vi "RILIS Remote Control.vi"() -> ()   [LabVIEW 2013]
uses:
  Global Variables/Global Stop.vi
panel:
  in  "Open Setup Scanner":bool
  in  "Step Size":i32=100 caption="Max. 500"
  in  "Enable Keyboard Control Button":bool
  in  "Open Scan Coordinator":bool
  in  "Tab Control":T1(tab)
  in  "Display History":i32=500 caption="Values"
  out "NB-TiSa Data vs Time":cluster{cluster{dbl, "Value":dbl}[]}[](graph)
  in  "Clear Time Graph":bool
  out "Wavelength vs. Thick Etalon Position":cluster{cluster{"Value":i32, "Value":dbl}[]}[](graph)
  out "Wavelength vs. Thin Etalon Position":cluster{cluster{"Value":i32, "Value":dbl}[]}[](graph)
  in  "Clear WL vs ThinPos":bool
  out "Power vs. Thick Etalon Position":cluster{cluster{"Value":i32, "Value":dbl}[]}[](graph)
  in  "Clear POW vs ThickPos":bool
  out "Power vs. Thin Etalon Position":cluster{cluster{"Value":i32, "Value":dbl}[]}[](graph)
  in  "Clear POW vs ThinPos":bool
  in  "Clear WL vs ThickPos":bool
  out "WS7 Pattern2 Data":u16[](graph)
  out "WS7 Pattern1 Data":u16[](graph)
  out "DAQ loop counter":i32
  out "Event Loop Counter":i32
  in  "Copy Values":bool
  in  "HELP Button":bool
  in  "Open Linewidth Sweep":bool
  in  "Open Dual Etalon Scanner":bool
  in  "Open Prop Stabilization":bool
  out "Thin Etalon Position":i32
  out "Thick Etalon Position":i32
  in  "Thin Etalon Position Setpoint":i32
  in  "Thick Etalon Position Setpoint":i32
  out "Linewidth":dbl format="%.2f"
  out "Power":dbl format="%.2f"
  in  "Stop":bool
  out "Wavenumber":dbl format="%.4f"
  # "UP, DOWN moves thick etalon\nLEFT, RIGHT moves thin etalon"
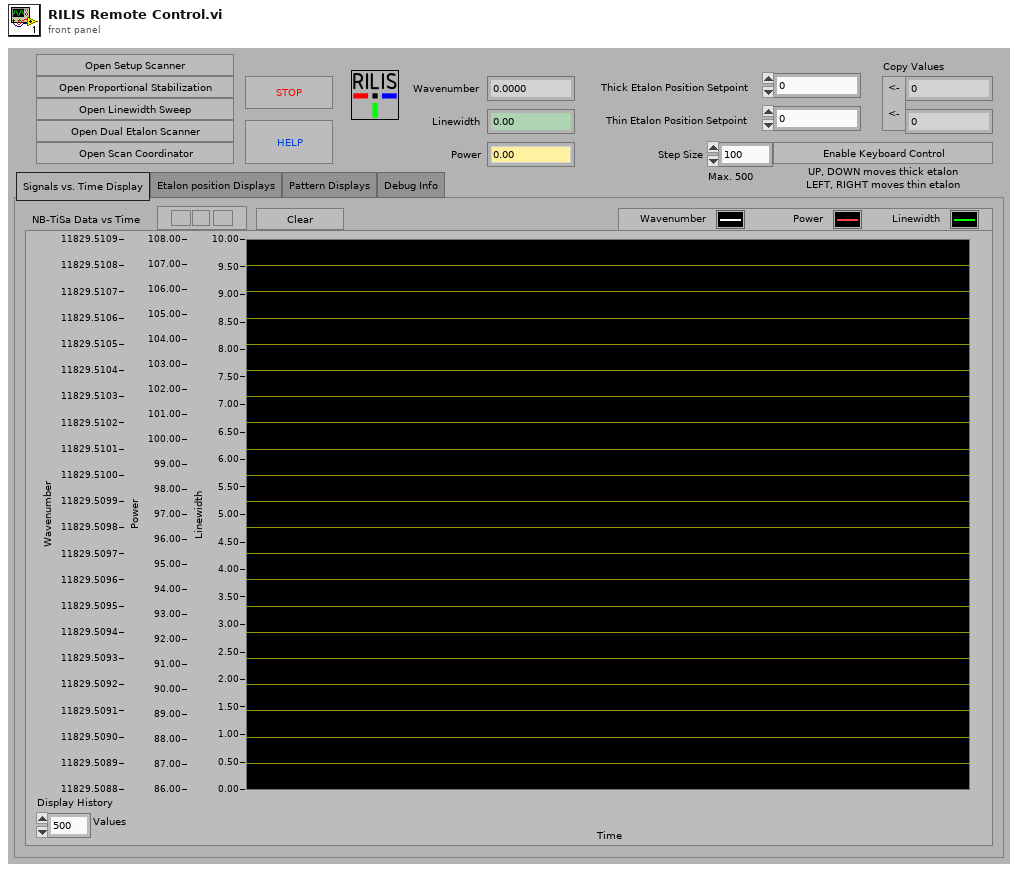
[diagram p1: front panel]
types:
  T1 = enum32{"Signals vs. Time Display", "Etalon position Displays", "Pattern Displays", "Debug Info"}
  T2 = enum32{"Bad", "Idle", "Run top level", "Running"}
  T3 = enum32{"Invalid", "Standard", "Closed", "Hidden", "Minimized", "Maximized"}
  T4 = typedef "eventvkey.ctl" = enum16{"ASCII", "Enter", "Return", "Shift", "Ctrl", "Alt", "Cmd", "Opt", "Caps", "NumLock", "Clear", "Break", "Up", "Down", "Left", "Right", "Insert", "Delete", "Home", "End", "PageUp", "PageDown", "Escape", "Help", "Pause", "ScrollLock", "F1", "F2", "F3", "F4", "F5", "F6", "F7", "F8", "F9", "F10", "F11", "F12", "F13", "F14", "F15", "F16", "F17", "F18", "F19", "F20", "F21", "F22", "F23", "F24", "Play", "VolumeUp", "VolumeDown", "Mute", "Two Byte Char"}
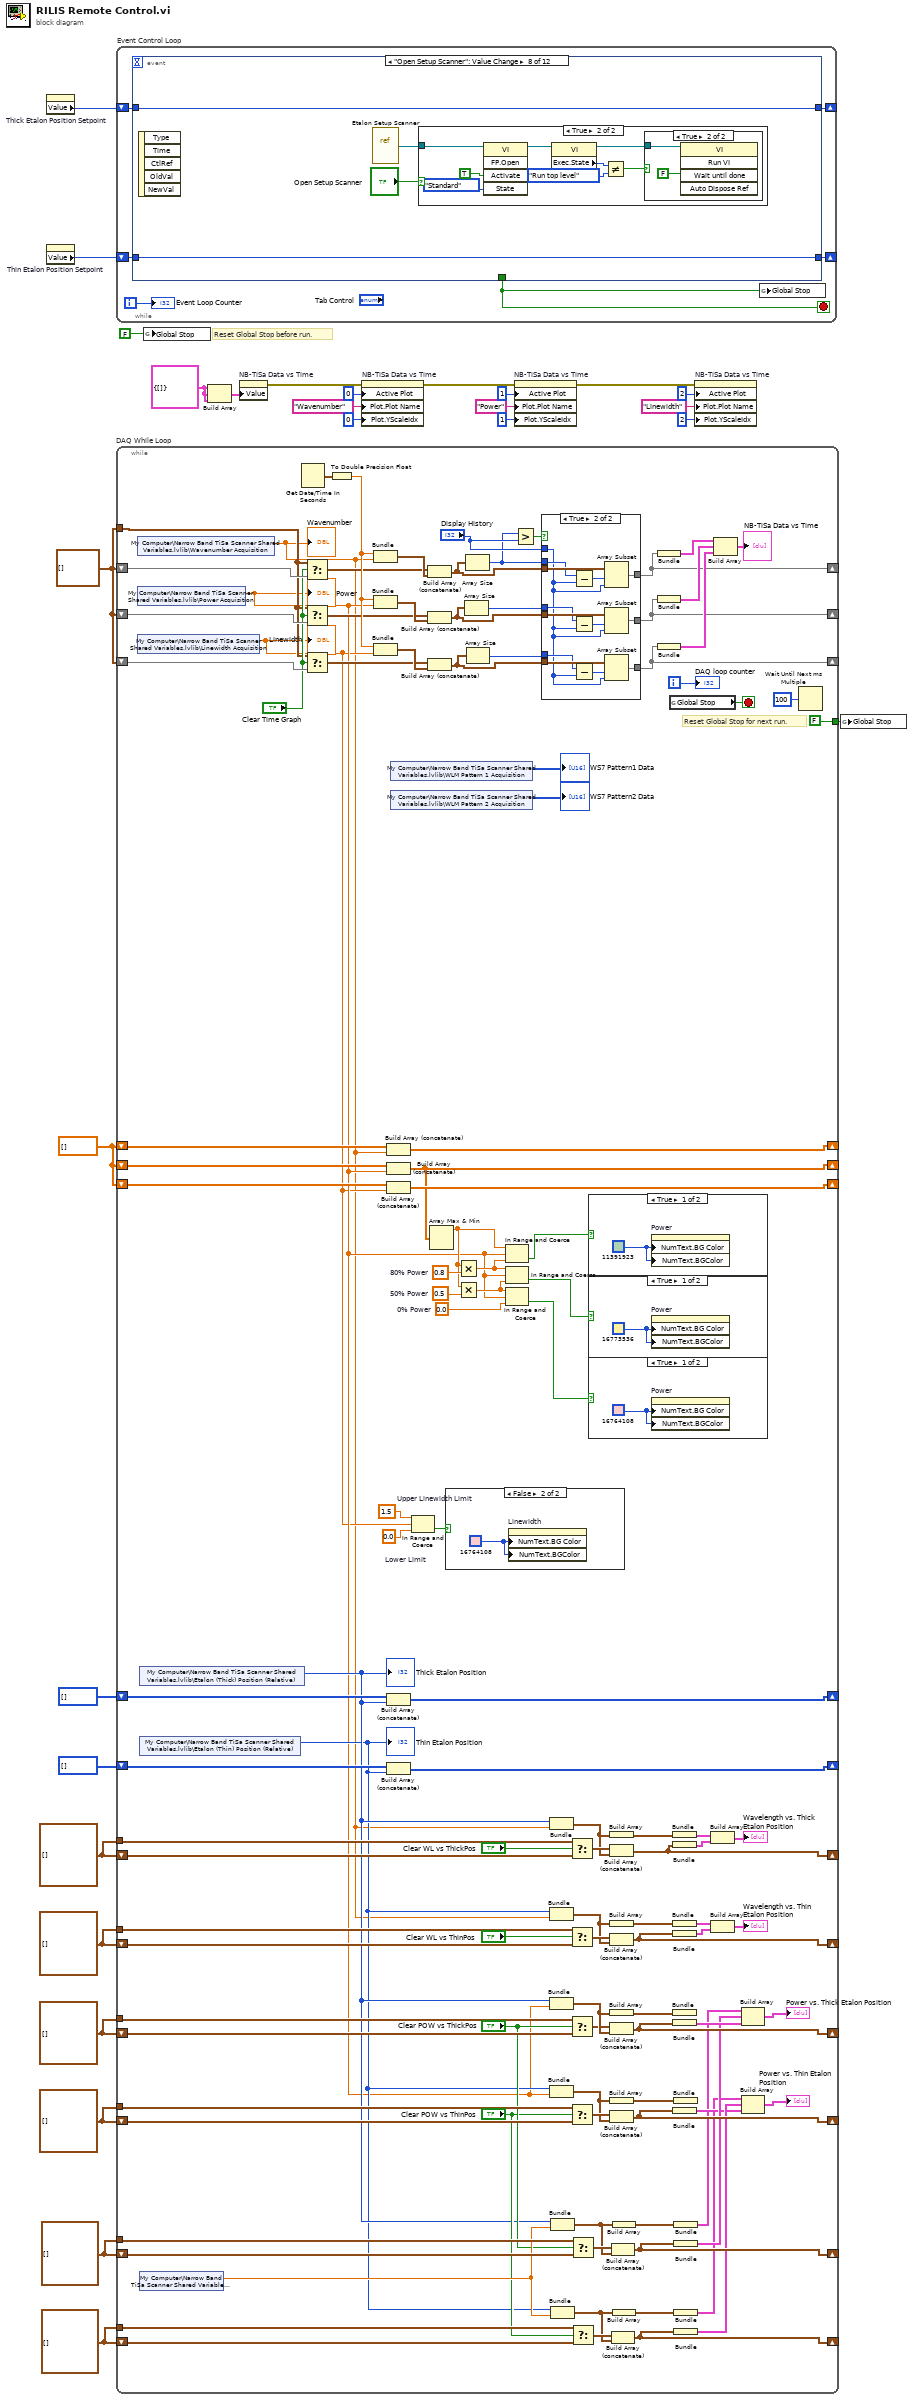
[diagram p0: block diagram]
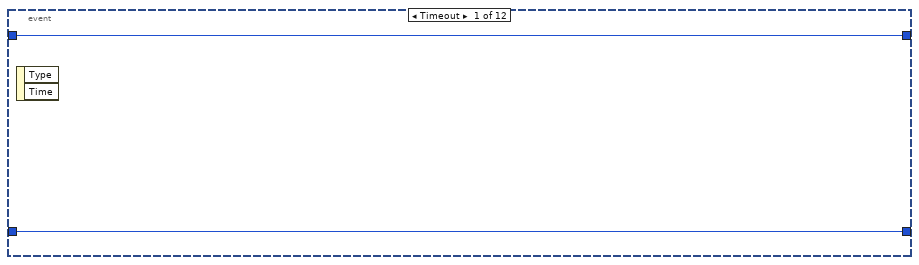
[diagram p2: hidden frame]
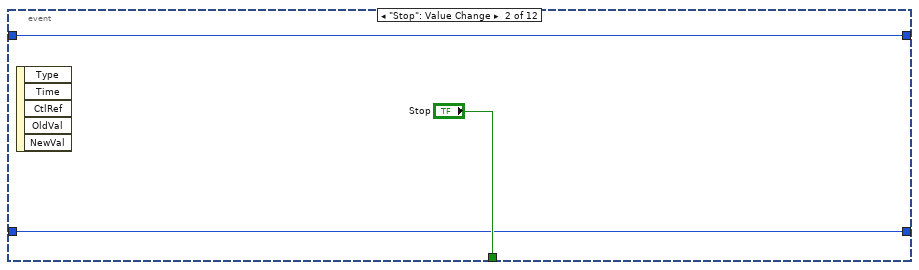
[diagram p3: hidden frame]
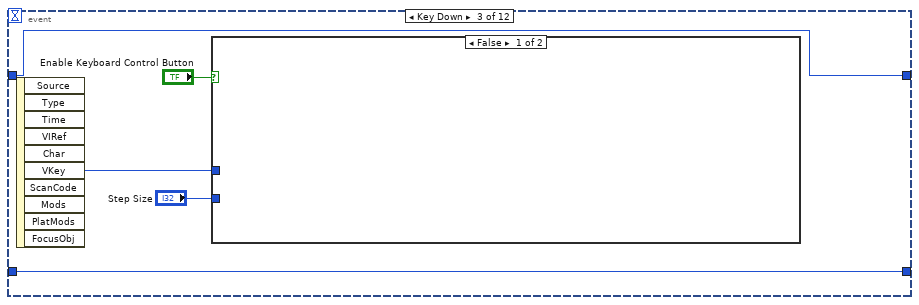
[diagram p4: hidden frame]
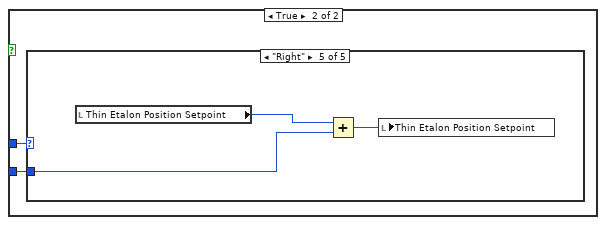
[diagram p5: hidden frame]
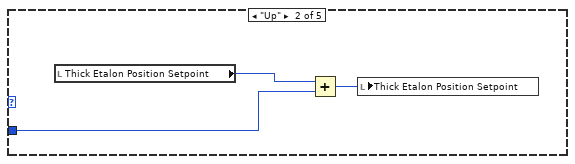
[diagram p7: hidden frame]
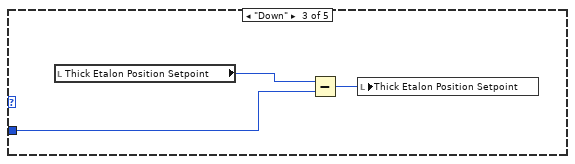
[diagram p8: hidden frame]
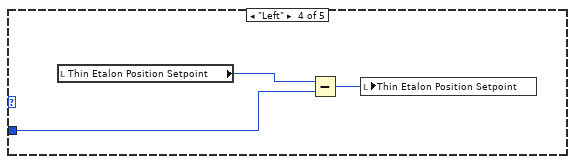
[diagram p9: hidden frame]
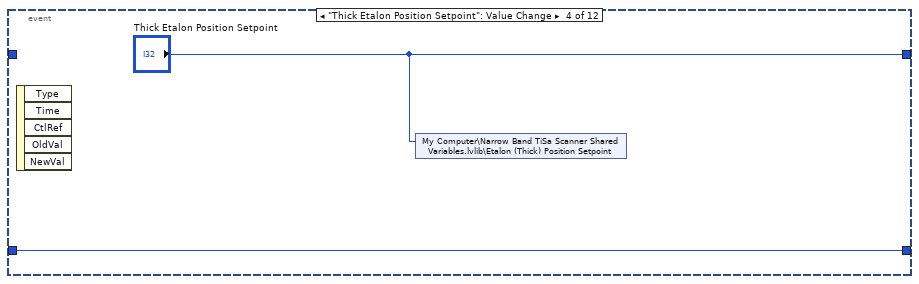
[diagram p10: hidden frame]
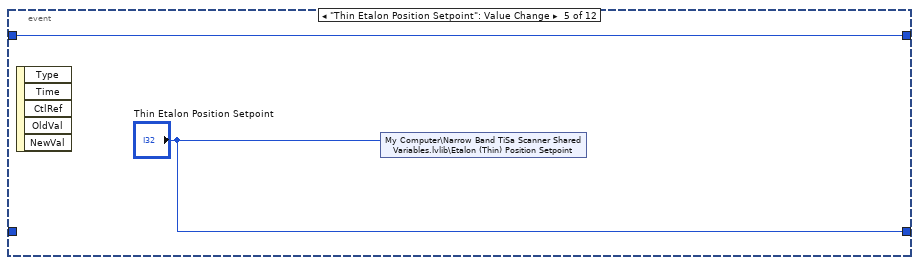
[diagram p11: hidden frame]
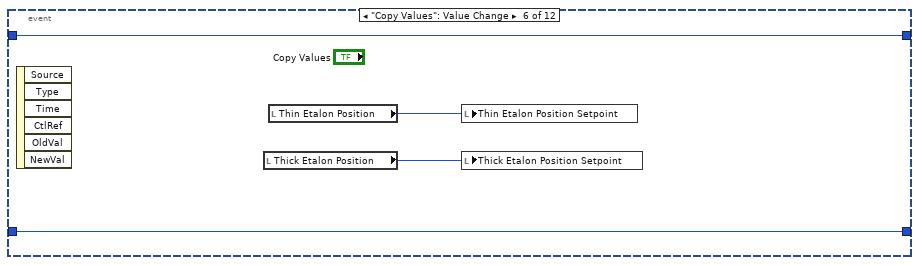
[diagram p12: hidden frame]
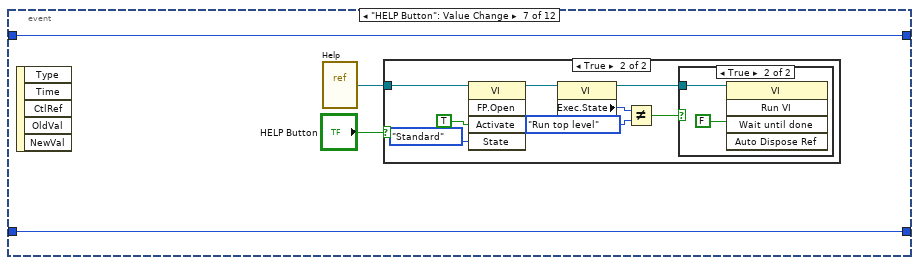
[diagram p13: hidden frame]
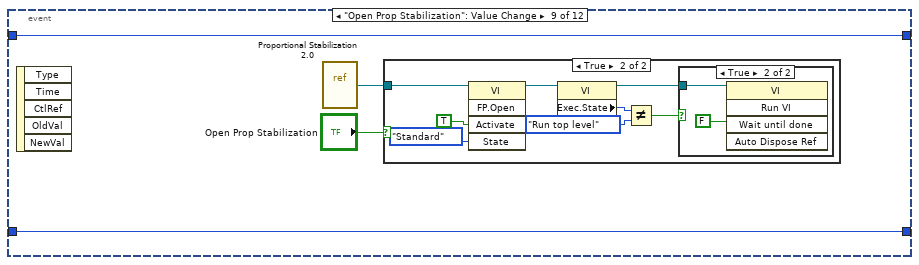
[diagram p18: hidden frame]
diagram:
  w2 = cluster{"Value":i32, "Value":dbl}[] []
  w1 = cluster{"Value":i32, "Value":dbl}[] []
  w3 = dbl[] []
  w6 = cluster{"Value":i32, "Value":dbl}[] []
  w7 = cluster{"Value":i32, "Value":dbl}[] []
  w8 = cluster{"Value":i32, "Value":dbl}[] []
  w9 = cluster{"Value":i32, "Value":dbl}[] []
  w27 = cluster{cluster{dbl, "Value":dbl}[]} {[]} ("output cluster")
  w12 = cluster{dbl, "Value":dbl}[] []
  # "Reset Global Stop before run."
  n1 = property on="Thick Etalon Position Setpoint" class="DigNum (strict)"() -> ("Value"=w11:i32)  [unwired: 2 in, 2 out]
  n2 = property on="Thin Etalon Position Setpoint" class="DigNum (strict)"() -> ("Value"=w10:i32)  [unwired: 2 in, 2 out]
  n3 = while "DAQ While Loop" {
    shift-right: [w130] -> _
    shift-left: w12 -> [w115]
    shift-right: [w129] -> _
    shift-left: w12 -> [w116]
    shift-right: [w128] -> _
    shift-left: w12 -> [w117]
    tunnel: [FALSE] -> w13
    tunnel: w12 -> [w113]
    shift-right: [w109] -> _
    shift-left: w9 -> [w111]
    shift-right: [w101] -> _
    shift-left: w8 -> [w103]
    tunnel: w9 -> [w105]
    tunnel: w8 -> [w104]
    shift-right: [w93] -> _
    shift-left: w7 -> [w91]
    tunnel: w7 -> [w90]
    shift-right: [w86] -> _
    shift-left: w6 -> [w88]
    tunnel: w6 -> [w89]
    shift-right: [w79] -> _
    shift-left: i32[] [] -> [w82]
    shift-right: [w78] -> _
    shift-left: i32[] [] -> [w81]
    shift-right: [w77] -> _
    shift-left: w3 -> [w80]
    shift-right: [w72] -> _
    shift-left: w3 -> [w71]
    shift-right: [w69] -> _
    shift-left: w3 -> [w70]
    shift-right: [w49] -> _
    shift-left: w1 -> [w51]
    tunnel: w1 -> [w52]
    shift-right: [w56] -> _
    shift-left: w2 -> [w54]
    tunnel: w2 -> [w53]
    i -> [w144]
    stop <- w122 stop-if-true
    w60 = 0.0  # 0% Power
    w63 = 0.5  # 50% Power
    w66 = 0.0  # Lower Limit
    w68 = 0.8  # 80% Power
    w67 = 1.5  # Upper Linewidth Limit
    # "Reset Global Stop for next run."
    n4 = shared-variable "My Computer\\Narrow Band TiSa Scanner Shared Variables.lvlib\\Wavenumber Acquisition"() -> (w29:dbl)  [unwired: 1 in, 1 out]
    "Wavenumber" <- w29
    n5 = shared-variable "My Computer\\Narrow Band TiSa Scanner Shared Variables.lvlib\\Power Acquisition"() -> (w43:dbl)  [unwired: 1 in, 1 out]
    "Power" <- w43
    n6 = shared-variable "My Computer\\Narrow Band TiSa Scanner Shared Variables.lvlib\\Linewidth Acquisition"() -> (w42:dbl)  [unwired: 1 in, 1 out]
    "Linewidth" <- w42
    n7 = shared-variable "My Computer\\Narrow Band TiSa Scanner Shared Variables.lvlib\\Etalon (Thick) Position (Relative)"() -> (w45:i32)  [unwired: 1 in, 1 out]
    "Thick Etalon Position" <- w45
    n8 = shared-variable "My Computer\\Narrow Band TiSa Scanner Shared Variables.lvlib\\Etalon (Thin) Position (Relative)"() -> (w44:i32)  [unwired: 1 in, 1 out]
    "Thin Etalon Position" <- w44
    n9 = shared-variable "My Computer\\Narrow Band TiSa Scanner Shared Variables.lvlib\\Power MPM"() -> (w48:dbl)  [unwired: 1 in, 1 out]
    n10 = Get Date/Time In Seconds() -> (seconds since 1Jan1904=w142:timestamp)
    n11 = Select(t=w113, s="Clear Time Graph", f=w115) -> (s? t:f=w120:cluster{dbl, "Double":dbl}[])
    n12 = Select(t=w113, s="Clear Time Graph", f=w116) -> (s? t:f=w119:cluster{dbl, "Double":dbl}[])
    n13 = Select(t=w113, s="Clear Time Graph", f=w117) -> (s? t:f=w118:cluster{dbl, "Double":dbl}[])
    n14 = To Double Precision Float(number=w142) -> (double precision float=w141:dbl)
    n15 = Bundle(w141, "Double"=w29) -> (w140:cluster{dbl, "Double":dbl})  [unwired: 1 in]
    n16 = Bundle(w141, "Double"=w43) -> (w139:cluster{dbl, "Double":dbl})  [unwired: 1 in]
    n17 = Bundle(w141, "Double"=w42) -> (w138:cluster{dbl, "Double":dbl})  [unwired: 1 in]
    n18 = Build Array (concatenate)(w80, w29) -> (w77:dbl[])
    n19 = Build Array (concatenate)(w70, w43) -> (w69:dbl[])
    n20 = Build Array (concatenate)(w71, w42) -> (w72:dbl[])
    n21 = Build Array (concatenate)(w82, w45) -> (w79:i32[])
    n22 = Build Array (concatenate)(w81, w44) -> (w78:i32[])
    n23 = shared-variable "My Computer\\Narrow Band TiSa Scanner Shared Variables.lvlib\\WLM Pattern 1 Acquisition"() -> (→"WS7 Pattern1 Data":u16[])  [unwired: 1 in, 1 out]
    n24 = shared-variable "My Computer\\Narrow Band TiSa Scanner Shared Variables.lvlib\\WLM Pattern 2 Acquisition"() -> (→"WS7 Pattern2 Data":u16[])  [unwired: 1 in, 1 out]
    n25 = In Range and Coerce(upper limit=w67, x=w42, lower limit=w66) -> (In Range?=w65:bool)  [unwired: 1 out]
    n26 = Build Array (concatenate)(w120, w140) -> (w132:cluster{dbl, "Double":dbl}[])
    n27 = Build Array (concatenate)(w119, w139) -> (w133:cluster{dbl, "Double":dbl}[])
    n28 = Build Array (concatenate)(w118, w138) -> (w131:cluster{dbl, "Double":dbl}[])
    n29 = Array Max & Min(array=w69) -> (max value=w62:dbl)  [unwired: 3 out]
    n30 = case shown="False" w65 {
      frame True {
        w148 = u32 11391923
        n31 = property on="Linewidth" class="DigNum (strict)"("NumText.BG Color"=w148, "NumText.BGColor"=w148) -> ()  [unwired: 2 in, 2 out]
      }
      frame False {
        w149 = u32 16764108
        n32 = property on="Linewidth" class="DigNum (strict)"("NumText.BG Color"=w149, "NumText.BGColor"=w149) -> ()  [unwired: 2 in, 2 out]
      }
    }
    n33 = Multiply(x=w62, y=w68) -> (x*y=w64:dbl)
    n34 = Multiply(x=w62, y=w63) -> (x*y=w61:dbl)
    n35 = Array Size(array=w133) -> (size(s)=w125:i32)
    n36 = Array Size(array=w132) -> (size(s)=w124:i32)
    n37 = Array Size(array=w131) -> (size(s)=w123:i32)
    n38 = In Range and Coerce(upper limit=w62, x=w43, lower limit=w64) -> (In Range?=w59:bool)  [unwired: 1 out]
    n39 = In Range and Coerce(upper limit=w64, x=w43, lower limit=w61) -> (In Range?=w58:bool)  [unwired: 1 out]
    n40 = In Range and Coerce(upper limit=w61, x=w43, lower limit=w60) -> (In Range?=w57:bool)  [unwired: 1 out]
    n41 = Greater?(x=w124, y="Display History") -> (0:w126:bool)
    n42 = case shown="True" w126 {
      tunnel: w133 -> [w151 w165]
      tunnel: w132 -> [w152 w164]
      tunnel: w131 -> [w150 w163]
      tunnel: [w152 w162] -> w130
      tunnel: [w151 w161] -> w129
      tunnel: [w150 w160] -> w128
      tunnel: "Display History" -> [_ w153]
      tunnel: w125 -> [_ w155]
      tunnel: w123 -> [_ w154]
      tunnel: w124 -> [_ w156]
      frame False {
      }
      frame True {
        n43 = Subtract(x=w156, y=w153) -> (x-y=w159:i32)
        n44 = Subtract(x=w155, y=w153) -> (x-y=w157:i32)
        n45 = Subtract(x=w154, y=w153) -> (x-y=w158:i32)
        n46 = Array Subset(array=w164, index=w159, length=w153) -> (w162:cluster{dbl, "Double":dbl}[])
        n47 = Array Subset(array=w165, index=w157, length=w153) -> (w161:cluster{dbl, "Double":dbl}[])
        n48 = Array Subset(array=w163, index=w158, length=w153) -> (w160:cluster{dbl, "Double":dbl}[])
      }
    }
    n49 = Bundle("Int32"=w45, "Double"=w29) -> (w108:cluster{"Int32":i32, "Double":dbl})  [unwired: 1 in]
    n50 = Bundle("Int32"=w44, "Double"=w29) -> (w100:cluster{"Int32":i32, "Double":dbl})  [unwired: 1 in]
    n51 = Bundle("Int32"=w45, "Double"=w43) -> (w94:cluster{"Int32":i32, "Double":dbl})  [unwired: 1 in]
    n52 = Bundle("Int32"=w44, "Double"=w43) -> (w85:cluster{"Int32":i32, "Double":dbl})  [unwired: 1 in]
    n53 = Bundle("Int32"=w45, "Double"=w48) -> (w34:cluster{"Int32":i32, "Double":dbl})  [unwired: 1 in]
    n54 = Bundle("Int32"=w44, "Double"=w48) -> (w35:cluster{"Int32":i32, "Double":dbl})  [unwired: 1 in]
    n55 = Select(t=w105, s="Clear WL vs ThickPos", f=w111) -> (s? t:f=w110:cluster{"Int32":i32, "Double":dbl}[])
    n56 = Select(t=w104, s="Clear WL vs ThinPos", f=w103) -> (s? t:f=w102:cluster{"Int32":i32, "Double":dbl}[])
    n57 = Select(t=w90, s="Clear POW vs ThickPos", f=w91) -> (s? t:f=w92:cluster{"Int32":i32, "Double":dbl}[])
    n58 = Select(t=w89, s="Clear POW vs ThinPos", f=w88) -> (s? t:f=w87:cluster{"Int32":i32, "Double":dbl}[])
    n59 = Select(t=w52, s="Clear POW vs ThickPos", f=w51) -> (s? t:f=w50:cluster{"Int32":i32, "Double":dbl}[])
    n60 = Select(t=w53, s="Clear POW vs ThinPos", f=w54) -> (s? t:f=w55:cluster{"Int32":i32, "Double":dbl}[])
    n61 = case shown="True" w59 {
      frame True {
        w147 = u32 11391923
        n62 = property on="Power" class="DigNum (strict)"("NumText.BG Color"=w147, "NumText.BGColor"=w147) -> ()  [unwired: 2 in, 2 out]
      }
      frame False {
      }
    }
    n63 = case shown="True" w58 {
      frame True {
        w146 = u32 16773536
        n64 = property on="Power" class="DigNum (strict)"("NumText.BG Color"=w146, "NumText.BGColor"=w146) -> ()  [unwired: 2 in, 2 out]
      }
      frame False {
      }
    }
    n65 = case shown="True" w57 {
      frame True {
        w145 = u32 16764108
        n66 = property on="Power" class="DigNum (strict)"("NumText.BG Color"=w145, "NumText.BGColor"=w145) -> ()  [unwired: 2 in, 2 out]
      }
      frame False {
      }
    }
    n67 = Build Array(w108) -> (w107:cluster{"Int32":i32, "Double":dbl}[])
    n68 = Build Array (concatenate)(w110, w108) -> (w109:cluster{"Int32":i32, "Double":dbl}[])
    n69 = Build Array(w100) -> (w99:cluster{"Int32":i32, "Double":dbl}[])
    n70 = Build Array (concatenate)(w102, w100) -> (w101:cluster{"Int32":i32, "Double":dbl}[])
    n71 = Build Array(w94) -> (w95:cluster{"Int32":i32, "Double":dbl}[])
    n72 = Build Array (concatenate)(w92, w94) -> (w93:cluster{"Int32":i32, "Double":dbl}[])
    n73 = Build Array(w85) -> (w84:cluster{"Int32":i32, "Double":dbl}[])
    n74 = Build Array (concatenate)(w87, w85) -> (w86:cluster{"Int32":i32, "Double":dbl}[])
    n75 = Build Array (concatenate)(w50, w34) -> (w49:cluster{"Int32":i32, "Double":dbl}[])
    n76 = Build Array (concatenate)(w55, w35) -> (w56:cluster{"Int32":i32, "Double":dbl}[])
    n77 = Build Array(w34) -> (w32:cluster{"Int32":i32, "Double":dbl}[])
    n78 = Build Array(w35) -> (w33:cluster{"Int32":i32, "Double":dbl}[])
    n79 = Bundle(w130) -> (w137:cluster{cluster{dbl, "Double":dbl}[]})  [unwired: 1 in]
    n80 = Bundle(w129) -> (w136:cluster{cluster{dbl, "Double":dbl}[]})  [unwired: 1 in]
    n81 = Bundle(w128) -> (w135:cluster{cluster{dbl, "Double":dbl}[]})  [unwired: 1 in]
    n82 = global read "Global Stop.vi" "Global Stop"() -> (w122:bool)
    n83 = Bundle(w107) -> (w75:cluster{cluster{"Int32":i32, "Double":dbl}[]})  [unwired: 1 in]
    n84 = Bundle(w109) -> (w76:cluster{cluster{"Int32":i32, "Double":dbl}[]})  [unwired: 1 in]
    n85 = Bundle(w99) -> (w73:cluster{cluster{"Int32":i32, "Double":dbl}[]})  [unwired: 1 in]
    n86 = Bundle(w101) -> (w74:cluster{cluster{"Int32":i32, "Double":dbl}[]})  [unwired: 1 in]
    n87 = Bundle(w95) -> ()  [unwired: 1 in, 1 out]
    n88 = Bundle(w93) -> (w39:cluster{cluster{"Int32":i32, "Double":dbl}[]})  [unwired: 1 in]
    n89 = Bundle(w86) -> (w36:cluster{cluster{"Int32":i32, "Double":dbl}[]})  [unwired: 1 in]
    n90 = Bundle(w84) -> ()  [unwired: 1 in, 1 out]
    n91 = Bundle(w32) -> (w30:cluster{cluster{"Int32":i32, "Double":dbl}[]})  [unwired: 1 in]
    n92 = Bundle(w49) -> (w38:cluster{cluster{"Int32":i32, "Double":dbl}[]})  [unwired: 1 in]
    n93 = Bundle(w33) -> (w31:cluster{cluster{"Int32":i32, "Double":dbl}[]})  [unwired: 1 in]
    n94 = Bundle(w56) -> (w37:cluster{cluster{"Int32":i32, "Double":dbl}[]})  [unwired: 1 in]
    n95 = Build Array(w75, w76) -> (→"Wavelength vs. Thick Etalon Position":cluster{cluster{"Int32":i32, "Double":dbl}[]}[])
    n96 = Build Array(w73, w74) -> (→"Wavelength vs. Thin Etalon Position":cluster{cluster{"Int32":i32, "Double":dbl}[]}[])
    n97 = Build Array(w137, w136, w135) -> (→"NB-TiSa Data vs Time":cluster{cluster{dbl, "Double":dbl}[]}[])
    n98 = Build Array(w30, w38, w39) -> (→"Power vs. Thick Etalon Position":cluster{cluster{"Int32":i32, "Double":dbl}[]}[])
    n99 = Build Array(w31, w37, w36) -> (→"Power vs. Thin Etalon Position":cluster{cluster{"Int32":i32, "Double":dbl}[]}[])
    n100 = Wait Until Next ms Multiple(millisecond multiple=u32 100) -> ()  [unwired: 1 out]
    "DAQ loop counter" <- w144
  }
  n101 = while "Event Control Loop" {
    shift-right: [w168] -> _
    shift-left: w11 -> [w169]
    shift-right: [w166] -> _
    shift-left: w10 -> [w167]
    i -> [w170]
    stop <- w171 stop-if-true
    n102 = event shown="[7] \"Open Setup Scanner\": Value Change" {
      selector: _ -> [_ _ _ _ _ _ _ _ _ _ _ _]
      dyn-events: _ -> [_ _ _ _ _ _ _ _ _ _ _ _]
      timeout: _ -> [_ _ _ _ _ _ _ _ _ _ _ _]
      tunnel: [_ "Stop" _ _ _ _ _ _ _ _ _ _] -> w171
      tunnel: w169 -> [w173 w175 w181 _ w199 w201 w206 w220 w233 w247 w262 w275]
      tunnel: [w173 w175 w181 "Thick Etalon Position Setpoint" w199 w201 w206 w220 w233 w247 w262 w275] -> w168
      tunnel: w167 -> [w172 w174 w180 w196 _ w200 w205 w219 w232 w246 w261 w274]
      tunnel: [w172 w174 w180 w196 "Thin Etalon Position Setpoint" w200 w205 w219 w232 w246 w261 w274] -> w166
      event Timeout {
        n103 = event-data() -> ()  [unwired: 1 in, 2 out]
      }
      event "Stop": Value Change {
        n104 = event-data() -> ()  [unwired: 1 in, 5 out]
      }
      event Key Down {
        n105 = event-data() -> ("VKey"=w179:T4)  [unwired: 1 in, 9 out]
        n106 = case shown="False" "Enable Keyboard Control Button" {
          tunnel: w179 -> [_ w183]
          tunnel: "Step Size" -> [_ w182]
          frame False {
          }
          frame True {
            n107 = case shown="\"Right\"" w183 {
              tunnel: w182 -> [_ w185 w188 w191 w194]
              frame "ASCII", Default {
              }
              frame "Up" {
                n108 = local read "Thick Etalon Position Setpoint"() -> (w186:i32)
                n109 = Add(x=w186, y=w185) -> (x+y=w184:i32)
                n110 = local write "Thick Etalon Position Setpoint"(w184) -> ()
              }
              frame "Down" {
                n111 = local read "Thick Etalon Position Setpoint"() -> (w189:i32)
                n112 = Subtract(x=w189, y=w188) -> (x-y=w187:i32)
                n113 = local write "Thick Etalon Position Setpoint"(w187) -> ()
              }
              frame "Left" {
                n114 = local read "Thin Etalon Position Setpoint"() -> (w192:i32)
                n115 = Subtract(x=w192, y=w191) -> (x-y=w190:i32)
                n116 = local write "Thin Etalon Position Setpoint"(w190) -> ()
              }
              frame "Right" {
                n117 = local read "Thin Etalon Position Setpoint"() -> (w195:i32)
                n118 = Add(x=w195, y=w194) -> (x+y=w193:i32)
                n119 = local write "Thin Etalon Position Setpoint"(w193) -> ()
              }
            }
          }
        }
      }
      event "Thick Etalon Position Setpoint": Value Change {
        n120 = event-data() -> ()  [unwired: 1 in, 5 out]
        n121 = shared-variable "My Computer\\Narrow Band TiSa Scanner Shared Variables.lvlib\\Etalon (Thick) Position Setpoint"("Thick Etalon Position Setpoint") -> ()  [unwired: 1 in, 1 out]
      }
      event "Thin Etalon Position Setpoint": Value Change {
        n122 = event-data() -> ()  [unwired: 1 in, 5 out]
        n123 = shared-variable "My Computer\\Narrow Band TiSa Scanner Shared Variables.lvlib\\Etalon (Thin) Position Setpoint"("Thin Etalon Position Setpoint") -> ()  [unwired: 1 in, 1 out]
      }
      event "Copy Values": Value Change {
        n124 = event-data() -> ()  [unwired: 1 in, 6 out]
        n125 = local read "Thick Etalon Position"() -> (w202:i32)
        n126 = local read "Thin Etalon Position"() -> (w203:i32)
        n127 = local write "Thin Etalon Position Setpoint"(w203) -> ()
        n128 = local write "Thick Etalon Position Setpoint"(w202) -> ()
      }
      event "HELP Button": Value Change {
        n129 = event-data() -> ()  [unwired: 1 in, 5 out]
        n130 = vi-ref "Help.vi"() -> (w207:refnum<vi>)
        n131 = case shown="True" "HELP Button" {
          tunnel: w207 -> [_ w208]
          frame False {
          }
          frame True {
            n132 = invoke class="VI" method="FP.Open"(reference=w208, "Activate"=TRUE ("Activate?"), "State"=T3."Standard") -> (reference out=w213:refnum<vi>)  [unwired: 2 in, 4 out]
            n133 = property class="VI"(reference=w213) -> (reference out=w212:refnum<vi>, "Exec.State"=w211:T2)  [unwired: 1 in, 1 out]
            n134 = Not Equal?(x=w211, y=T2."Run top level" ("Execution:State")) -> (x != y?=w209:bool)
            n135 = case shown="True" w209 {
              tunnel: w212 -> [_ w216]
              frame False {
              }
              frame True {
                n136 = invoke class="VI" method="Run VI"(reference=w216, "Wait until done"=FALSE ("Wait Until Done")) -> ()  [unwired: 3 in, 5 out]
              }
            }
          }
        }
      }
      event "Open Setup Scanner": Value Change {
        n137 = event-data() -> ()  [unwired: 1 in, 5 out]
        n138 = vi-ref "Etalon Setup Scanner.vi"() -> (w221:refnum<vi>)
        n139 = case shown="True" "Open Setup Scanner" {
          tunnel: w221 -> [_ w222]
          frame False {
          }
          frame True {
            n140 = invoke class="VI" method="FP.Open"(reference=w222, "Activate"=TRUE ("Activate?"), "State"=T3."Standard") -> (reference out=w227:refnum<vi>)  [unwired: 2 in, 4 out]
            n141 = property class="VI"(reference=w227) -> (reference out=w226:refnum<vi>, "Exec.State"=w225:T2)  [unwired: 1 in, 1 out]
            n142 = Not Equal?(x=w225, y=T2."Run top level" ("Execution:State")) -> (x != y?=w223:bool)
            n143 = case shown="True" w223 {
              tunnel: w226 -> [_ w230]
              frame False {
              }
              frame True {
                n144 = invoke class="VI" method="Run VI"(reference=w230, "Wait until done"=FALSE ("Wait Until Done")) -> ()  [unwired: 3 in, 5 out]
              }
            }
          }
        }
      }
      event "Open Prop Stabilization": Value Change {
        n145 = event-data() -> ()  [unwired: 1 in, 5 out]
        n146 = vi-ref "Proportional Stabilization 2.0.vi"() -> (w234:refnum<vi>)
        n147 = case shown="True" "Open Prop Stabilization" {
          tunnel: w234 -> [_ w236]
          frame False {
          }
          frame True {
            n148 = invoke class="VI" method="FP.Open"(reference=w236, "Activate"=TRUE ("Activate?"), "State"=T3."Standard") -> (reference out=w241:refnum<vi>)  [unwired: 2 in, 4 out]
            n149 = property class="VI"(reference=w241) -> (reference out=w240:refnum<vi>, "Exec.State"=w239:T2)  [unwired: 1 in, 1 out]
            n150 = Not Equal?(x=w239, y=T2."Run top level" ("Execution:State")) -> (x != y?=w237:bool)
            n151 = case shown="True" w237 {
              tunnel: w240 -> [_ w244]
              frame False {
              }
              frame True {
                n152 = invoke class="VI" method="Run VI"(reference=w244, "Wait until done"=FALSE ("Wait Until Done")) -> ()  [unwired: 3 in, 5 out]
              }
            }
          }
        }
      }
      event "Open Dual Etalon Scanner": Value Change {
        n153 = event-data() -> ()  [unwired: 1 in, 5 out]
        n154 = vi-ref "Dual Etalon Scanner.vi"() -> (w248:refnum<vi>)
        n155 = case shown="True" "Open Dual Etalon Scanner" {
          tunnel: w248 -> [_ w250]
          frame False {
          }
          frame True {
            n156 = invoke class="VI" method="FP.Open"(reference=w250, "Activate"=TRUE ("Activate?"), "State"=T3."Standard") -> (reference out=w255:refnum<vi>)  [unwired: 2 in, 4 out]
            n157 = property class="VI"(reference=w255) -> (reference out=w254:refnum<vi>, "Exec.State"=w253:T2)  [unwired: 1 in, 1 out]
            n158 = Not Equal?(x=w253, y=T2."Run top level" ("Execution:State")) -> (x != y?=w251:bool)
            n159 = case shown="True" w251 {
              tunnel: w254 -> [_ w258]
              frame False {
              }
              frame True {
                n160 = invoke class="VI" method="Run VI"(reference=w258, "Wait until done"=FALSE ("Wait Until Done")) -> ()  [unwired: 3 in, 5 out]
              }
            }
          }
        }
      }
      event "Open Scan Coordinator": Value Change {
        n161 = event-data() -> ()  [unwired: 1 in, 5 out]
        n162 = vi-ref "RILIS Narrow Band Scan Coordinator 2.0.vi"() -> (w263:refnum<vi>)
        n163 = case shown="True" "Open Scan Coordinator" {
          tunnel: w263 -> [_ w264]
          frame False {
          }
          frame True {
            n164 = invoke class="VI" method="FP.Open"(reference=w264, "Activate"=TRUE ("Activate?"), "State"=T3."Standard") -> (reference out=w269:refnum<vi>)  [unwired: 2 in, 4 out]
            n165 = property class="VI"(reference=w269) -> (reference out=w268:refnum<vi>, "Exec.State"=w267:T2)  [unwired: 1 in, 1 out]
            n166 = Not Equal?(x=w267, y=T2."Run top level" ("Execution:State")) -> (x != y?=w265:bool)
            n167 = case shown="True" w265 {
              tunnel: w268 -> [_ w272]
              frame False {
              }
              frame True {
                n168 = invoke class="VI" method="Run VI"(reference=w272, "Wait until done"=FALSE ("Wait Until Done")) -> ()  [unwired: 3 in, 5 out]
              }
            }
          }
        }
      }
      event "Open Linewidth Sweep": Value Change {
        n169 = event-data() -> ()  [unwired: 1 in, 5 out]
        n170 = vi-ref "Thin Etalon Linewidth Sweep 2.0 user.vi"() -> (w276:refnum<vi>)
        n171 = case shown="True" "Open Linewidth Sweep" {
          tunnel: w276 -> [_ w278]
          frame False {
          }
          frame True {
            n172 = invoke class="VI" method="FP.Open"(reference=w278, "Activate"=TRUE ("Activate?"), "State"=T3."Standard") -> (reference out=w283:refnum<vi>)  [unwired: 2 in, 4 out]
            n173 = property class="VI"(reference=w283) -> (reference out=w282:refnum<vi>, "Exec.State"=w281:T2)  [unwired: 1 in, 1 out]
            n174 = Not Equal?(x=w281, y=T2."Run top level" ("Execution:State")) -> (x != y?=w279:bool)
            n175 = case shown="True" w279 {
              tunnel: w282 -> [_ w286]
              frame False {
              }
              frame True {
                n176 = invoke class="VI" method="Run VI"(reference=w286, "Wait until done"=FALSE ("Wait Until Done")) -> ()  [unwired: 3 in, 5 out]
              }
            }
          }
        }
      }
    }
    n177 = global write "Global Stop.vi" "Global Stop"(w171) -> ()
    "Event Loop Counter" <- w170
  }
  n178 = global write "Global Stop.vi" "Global Stop"(FALSE) -> ()
  n179 = Build Array(w27, w27, w27) -> (w28:cluster{cluster{dbl, "Value":dbl}[]}[])
  n180 = property on="NB-TiSa Data vs Time" class="XYGraph (strict)"("Value"=w28) -> (error out=w26:errorcluster)  [unwired: 2 in, 1 out]
  n181 = property on="NB-TiSa Data vs Time" class="XYGraph (strict)"(error in=w26, "Active Plot"=u32 0, "Plot.Plot Name"="Wavenumber", "Plot.YScaleIdx"=u32 0 ("Plot.Y Scale Index")) -> (error out=w16:errorcluster)  [unwired: 1 in, 1 out]
  n182 = property on="NB-TiSa Data vs Time" class="XYGraph (strict)"(error in=w16, "Active Plot"=u32 1, "Plot.Plot Name"="Power", "Plot.YScaleIdx"=u32 1 ("Plot.Y Scale Index")) -> (error out=w15:errorcluster)  [unwired: 1 in, 1 out]
  n183 = property on="NB-TiSa Data vs Time" class="XYGraph (strict)"(error in=w15, "Active Plot"=u32 2, "Plot.Plot Name"="Linewidth", "Plot.YScaleIdx"=u32 2 ("Plot.Y Scale Index")) -> ()  [unwired: 1 in, 2 out]
  n184 = global write "Global Stop.vi" "Global Stop"(w13) -> ()
